vi "Find Valid Step.vi"(8 "error in (no error)":errorcluster, 10 "Starting Step":i32, 11 "Output Sequencer in":refnum<class "Output Sequencer.lvclass">) -> (0 "error out":errorcluster, 1 "Next Cycle?":bool, 2 "Next Step":i32, 3 "Output Sequencer out":refnum<class "Output Sequencer.lvclass">, 4 "Valid Step Found":bool)   [LabVIEW 2020, in "Output Sequencer.lvlib" / "Output Sequencer.lvclass"]
uses:
  Output Sequencer.lvclass
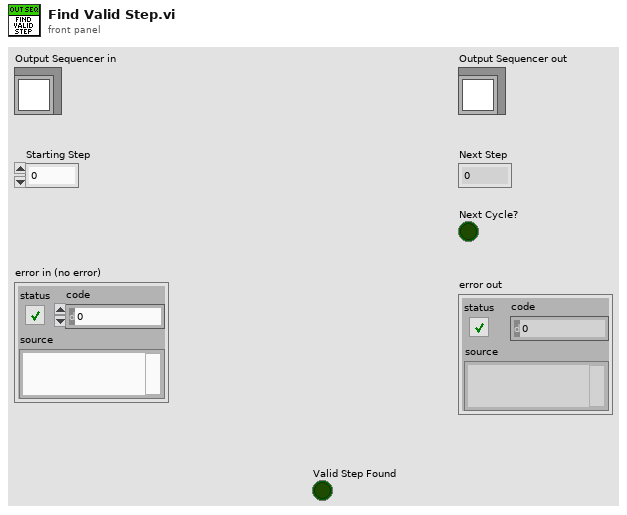
[diagram p1: front panel]
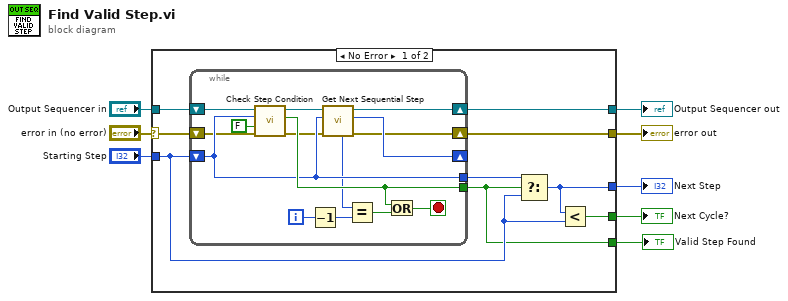
[diagram p0: block diagram]
diagram:
  n1 = case shown="No Error" "error in (no error)" {
    selector: "error in (no error)" -> [w9 w34]
    tunnel: [w17 _] -> w8
    tunnel: "Starting Step" -> [w16 _]
    tunnel: [w15 _] -> w6
    tunnel: "Output Sequencer in" -> [w14 w33]
    tunnel: [w13 w33] -> w4
    tunnel: [w11 _] -> w3
    tunnel: [w10 w34] -> w2
    frame No Error {
      n2 = while {
        shift-right: [w28] -> _
        shift-left: w16 -> [w26]
        tunnel: [w27] -> w15
        tunnel: [w26] -> w12
        shift-right: [w22] -> w13
        shift-left: w14 -> [w24]
        shift-right: [w18] -> w10
        shift-left: w9 -> [w19]
        i -> [w30]
        stop <- w32 stop-if-true
        n3 = call "Check Step Condition.vi"("error in (no error)"=w19, "Postcondition?"=FALSE, "Step Number"=w26, "Output Sequencer in"=w24) -> ("error out"=w20:errorcluster, "Condition passed"=w27:bool, "Output Sequencer out"=w23:refnum<class "Output Sequencer.lvclass">)  [unwired: 4 in, 1 out]
        n4 = Decrement(x=w30) -> (x-1=w29:i32)
        n5 = call "Get Next Sequential Step.vi"("error in (no error)"=w20, "Current Step"=w26, "Output Sequencer in"=w23) -> ("error out"=w18:errorcluster, "Next Step"=w28:i32, "Output Sequencer out"=w22:refnum<class "Output Sequencer.lvclass">, "Number of Steps"=w21:i32)  [unwired: 4 in, 1 out]
        n6 = Equal?(x=w21, y=w29) -> (x = y?=w31:bool)
        n7 = Or(x=w27, y=w31) -> (x .or. y?=w32:bool)
      }
      n8 = Select(t=w12, s=w15, f=w16) -> (s? t:f=w17:i32)
      n9 = Less?(x=w17, y=w16) -> (x < y?=w11:bool)
    }
    frame Error {
    }
  }
  "Next Step" <- w8
  "Next Cycle?" <- w3
  "Output Sequencer out" <- w4
  "Valid Step Found" <- w6
  "error out" <- w2
